vi "MPExxx Revision Query.vi"(0 "VISA session":refnum<visa-resource-name>, 1 "error in (no error)":errorcluster) -> (2 "dup VISA session":refnum<visa-resource-name>, 3 "instr driver revision":string, 4 "instr firmware revision":string, 5 "error out":errorcluster)   [LabVIEW 2012]
doc: "This VI queries the current instrument firmware revision and instrument driver revision.\n\nMagna-Power Electronics, Inc. DC Power Supply\nCreated By: Robert Limlaw\nRelease Date: 8/04\nVersion: 1.2\nOriginally Developed in LabVIEW Version: 6.0\n\nModification History: \n\nVersion 1.0\nInitial Release.\n\nVersion 1.1\nAdded PQA, SQA, MQA and MTA functionality to driver.\n\nVersion 1.2\nAdded modulation functionality to the PQD, SQD, MQD and MTD systems."
panel:
  # "MAGNA-POWER"
  # "Electronics"
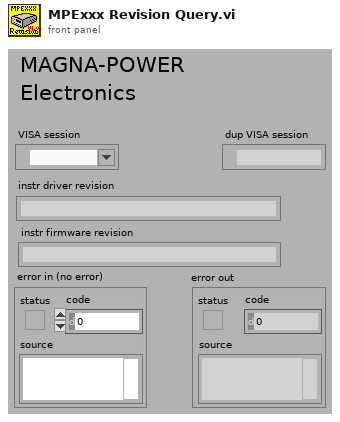
[diagram p1: front panel]
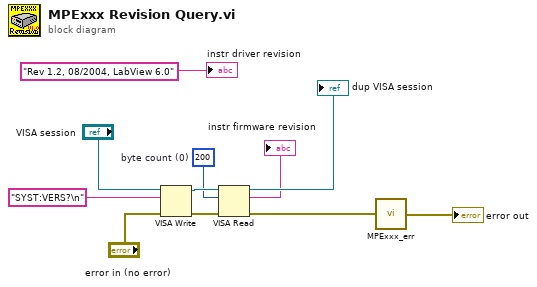
[diagram p0: block diagram]
diagram:
  w8 = u32 200  # byte count (0)
  n1 = VISA Write(VISA resource name="VISA session", write buffer="SYST:VERS?\n", error in (no error)="error in (no error)") -> (VISA resource name out=w9:refnum<visa-resource-name>, error out=w7:errorcluster)  [unwired: 1 out]
  n2 = VISA Read(VISA resource name=w9, byte count=w8, error in (no error)=w7) -> (VISA resource name out=→"dup VISA session":refnum<visa-resource-name>, read buffer=→"instr firmware revision":string, error out=w6:errorcluster)  [unwired: 1 out]
  n3 = call "MPExxx_err.vi"("error in (no error)"=w6) -> ("error out"=→"error out":errorcluster)
  "instr driver revision" <- "Rev 1.2, 08/2004, LabView 6.0"
